vi "Read Control Refnum.vi"(8 "error in (no error)":errorcluster, 11 "MCLB_Lib in":refnum<class "MCLB_Lib.lvclass">) -> (0 "error out":errorcluster, 2 "Control Refnum":refnum<vi>, 3 "MCLB_Lib out":refnum<class "MCLB_Lib.lvclass">)   [LabVIEW 2020, in "MCLB_Lib.lvclass"]
uses:
  MCLB_Lib.lvclass
  MCLB_Lib.lvclass/MCLB_Lib.ctl
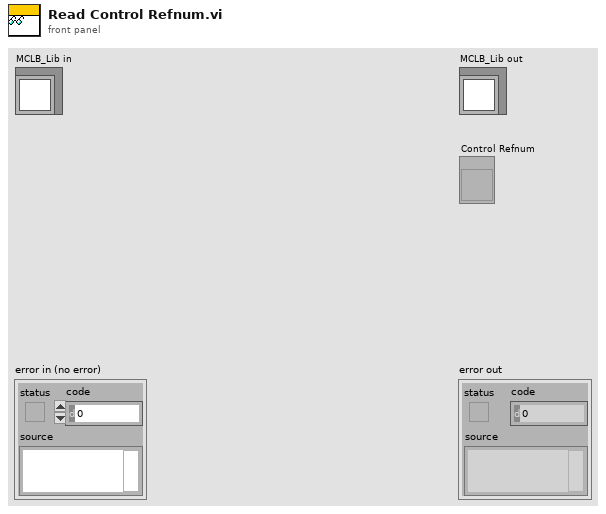
[diagram p1: front panel]
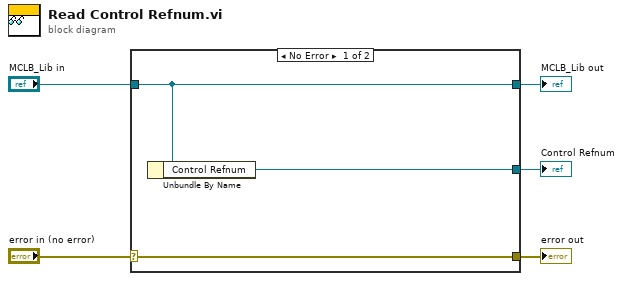
[diagram p0: block diagram]
diagram:
  n1 = case shown="No Error" "error in (no error)" {
    selector: "error in (no error)" -> [w8 w9]
    tunnel: [w8 w9] -> w4
    tunnel: [w7 w10] -> w2
    tunnel: "MCLB_Lib in" -> [w7 w10]
    tunnel: [w6 _] -> w1
    frame No Error {
      n2 = Unbundle By Name(w7) -> ("Control Refnum"=w6:refnum<vi>)
    }
    frame Error {
    }
  }
  "error out" <- w4
  "MCLB_Lib out" <- w2
  "Control Refnum" <- w1
